vi "logStartupChecks.vi"(8 "error in (no error)":errorcluster, 10 "EventStartupChecks":T1, 11 "M1M3SAL in":refnum<class "M1M3SAL.lvclass">) -> (0 "error out":errorcluster, 3 "M1M3SAL out":refnum<class "M1M3SAL.lvclass">)   [LabVIEW 2016, in "M1M3SupportCommunicator.lvlib" / "M1M3SAL.lvclass"]
uses:
  M1M3SAL.lvclass
  DataTypes/Topics/EventStartupChecks.ctl
  DataTypes/Topics/Parts/Timestamp.ctl
  DataTypes/MessageHeader.ctl
  DataTypes/MessageTypes.ctl
  DataTypes/MessageTopics.ctl
  Common_RT_Utilities/U8ArrayBuilderAutoIndexing/U8ArrayBuilderAutoIndexing.lvclass
  M1M3SupportCommunicator.lvlib
  DataTypes/Topics/M1M3SupportTopics.lvlib
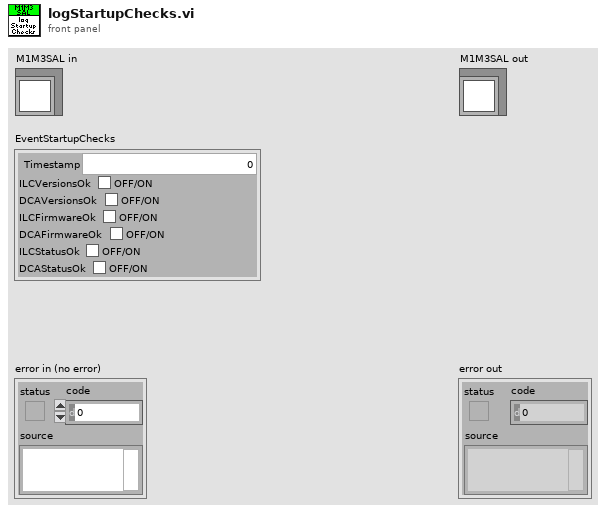
[diagram p1: front panel]
types:
  T1 = typedef "M1M3SupportTopics.lvlib/EventStartupChecks.ctl" = cluster{"Timestamp":T2, "ILCVersionsOk":bool, "DCAVersionsOk":bool, "ILCFirmwareOk":bool, "DCAFirmwareOk":bool, "ILCStatusOk":bool, "DCAStatusOk":bool}
  T2 = typedef "M1M3SupportTopics.lvlib/Timestamp.ctl" = dbl
  T3 = typedef "M1M3SupportCommunicator.lvlib/MessageHeader.ctl" = cluster{"Type":T4, "Topic":T5, "Size":i32}
  T4 = typedef "M1M3SupportCommunicator.lvlib/MessageTypes.ctl" = enum8{"None", "PutSample", "GetNextSample", "LogEvent", "GetEvent", "IssueCommand", "CommandId", "WaitForCompletion", "AcceptCommand", "AckCommand"}
  T5 = typedef "M1M3SupportCommunicator.lvlib/MessageTopics.ctl" = enum8{"None", "ForceActuatorData", "MirrorForceData", "HardpointData", "AirData", "DynamicData", "FPGAData", "IMSData", "ForceActuatorStatus", "ElevationData", "HardpointStatus", "HardpointActuatorChase", "AirStatus", "ForceActuatorSafetyChecks", "ForceActuatorTest", "ActuatorBroadcastCounter", "StatusChecks", "CellChecks", "HardpointActuatorBreakaway", "RaiseMirrorComplete", "ILCCommunication", "ElevationAngleChecks", "DetailedState", "ServoLoops", "ForceActuatorInfo", "LowerMirrorComplete", "HardpointActuatorInfo", "SettingsApplied", "ErrorCode", "StartupChecks", "SummaryState", "SettingVersions", "ActuatorTestStatus", "AppliedSettingsMatchStart", "Enable", "EnterMaintenance", "Standby", "AbortLowerM1M3", "ApplyAberrationByForces", "ApplyAOSCorrectionByBendingModes", "ClearAOSCorrection", "Start", "RaiseM1M3", "TestForceActuator", "LowerM1M3", "ApplyAOSCorrectionByForces", "Disable", "ApplyAberationByBendingMode", "TestHardpoint", "ManipulateM1M3", "ClearAberration", "Exit", "TestAir", "AbortRaiseM1M3", "MoveHardpointActuators", "ExitMaintenance", "Shutdown"}
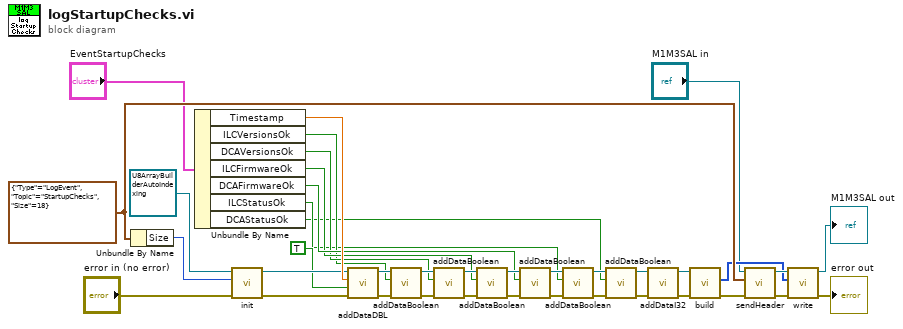
[diagram p0: block diagram]
diagram:
  w37 = T3 {"Type"=enum."LogEvent", "Topic"=enum."StartupChecks", "Size"=18} ("MessageHeader")
  n1 = Unbundle By Name(w37) -> ("Size"=w36:i32)
  n2 = Unbundle By Name("EventStartupChecks") -> ("Timestamp"=w27:T2, "ILCVersionsOk"=w12:bool, "DCAVersionsOk"=w13:bool, "ILCFirmwareOk"=w14:bool, "DCAFirmwareOk"=w15:bool, "ILCStatusOk"=w6:bool, "DCAStatusOk"=w5:bool)
  n3 = call "init.vi"("error in (no error)"="error in (no error)", "Size"=w36, "U8ArrayBuilderAutoIndexing in"=refnum<class "U8ArrayBuilderAutoIndexing.lvclass"> refnum ("RTUtilities.lvlib:U8ArrayBuilderAutoIndexing.lvclass")) -> ("error out"=w24:errorcluster, "U8ArrayBuilderAutoIndexing out"=w26:refnum<class "U8ArrayBuilderAutoIndexing.lvclass">)  [unwired: 7 in]
  n4 = call "addDataDBL.vi"("error in (no error)"=w24, "OverrideSwapBytes"=TRUE, "Data"=w27, "U8ArrayBuilderAutoIndexing in"=w26) -> ("error out"=w18:errorcluster, "U8ArrayBuilderAutoIndexing out"=w19:refnum<class "U8ArrayBuilderAutoIndexing.lvclass">)  [unwired: 6 in]
  n5 = call "addDataBoolean.vi"("error in (no error)"=w18, "Data"=w12, "U8ArrayBuilderAutoIndexing in"=w19) -> ("error out"=w23:errorcluster, "U8ArrayBuilderAutoIndexing out"=w22:refnum<class "U8ArrayBuilderAutoIndexing.lvclass">)  [unwired: 7 in]
  n6 = call "addDataBoolean.vi"("error in (no error)"=w23, "Data"=w13, "U8ArrayBuilderAutoIndexing in"=w22) -> ("error out"=w21:errorcluster, "U8ArrayBuilderAutoIndexing out"=w20:refnum<class "U8ArrayBuilderAutoIndexing.lvclass">)  [unwired: 7 in]
  n7 = call "addDataBoolean.vi"("error in (no error)"=w21, "Data"=w14, "U8ArrayBuilderAutoIndexing in"=w20) -> ("error out"=w17:errorcluster, "U8ArrayBuilderAutoIndexing out"=w16:refnum<class "U8ArrayBuilderAutoIndexing.lvclass">)  [unwired: 7 in]
  n8 = call "addDataBoolean.vi"("error in (no error)"=w17, "Data"=w15, "U8ArrayBuilderAutoIndexing in"=w16) -> ("error out"=w10:errorcluster, "U8ArrayBuilderAutoIndexing out"=w9:refnum<class "U8ArrayBuilderAutoIndexing.lvclass">)  [unwired: 7 in]
  n9 = call "addDataBoolean.vi"("error in (no error)"=w10, "Data"=w6, "U8ArrayBuilderAutoIndexing in"=w9) -> ("error out"=w8:errorcluster, "U8ArrayBuilderAutoIndexing out"=w7:refnum<class "U8ArrayBuilderAutoIndexing.lvclass">)  [unwired: 7 in]
  n10 = call "addDataBoolean.vi"("error in (no error)"=w8, "Data"=w5, "U8ArrayBuilderAutoIndexing in"=w7) -> ("error out"=w1:errorcluster, "U8ArrayBuilderAutoIndexing out"=w4:refnum<class "U8ArrayBuilderAutoIndexing.lvclass">)  [unwired: 7 in]
  n11 = call "addDataI32.vi"("error in (no error)"=w1, "U8ArrayBuilderAutoIndexing in"=w4) -> ("error out"=w2:errorcluster, "U8ArrayBuilderAutoIndexing out"=w3:refnum<class "U8ArrayBuilderAutoIndexing.lvclass">)  [unwired: 8 in]
  n12 = call "build.vi"("error in (no error)"=w2, "U8ArrayBuilderAutoIndexing in"=w3) -> ("error out"=w33:errorcluster, "Array"=w34:u8[])  [unwired: 7 in, 1 out]
  n13 = call "sendHeader.vi"("error in (no error)"=w33, "MessageHeader"=w37, "M1M3SAL in"="M1M3SAL in") -> ("error out"=w32:errorcluster, "M1M3SAL out"=w35:refnum<class "M1M3SAL.lvclass">)  [unwired: 7 in]
  n14 = call "write.vi"("error in (no error)"=w32, "Data"=w34, "M1M3SAL in"=w35) -> ("error out"=→"error out":errorcluster, "M1M3SAL out"=→"M1M3SAL out":refnum<class "M1M3SAL.lvclass">)  [unwired: 7 in]
